vi "BRig_dataBlock_nTrial.vi"() -> (2 "output_nTrial":i32)   [LabVIEW 2014]
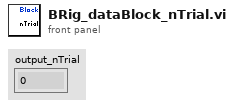
[diagram p1: front panel]
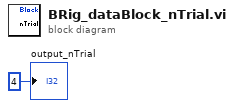
[diagram p0: block diagram]
diagram:
  "output_nTrial" <- 4 ("output_iBlock")
